vi "dosimat876_deliver.vi"(4 "error in":errorcluster, 6 "Volume":dbl format="%_4f", 7 "Dosimat Port In":refnum<visa-resource-name>="COM1") -> (0 "error out":errorcluster, 1 "Coerced?":bool, 2 "OutVolume":dbl, 3 "Dosimat Port Out":refnum<visa-resource-name>="COM1")   [LabVIEW 2010]
panel:
  # "Volume coerced!\nThe 876 will only accept volumes between 0.05 and 5.00 ml in increments of 0.05 ml. The volume has been changed to meet these requirements."
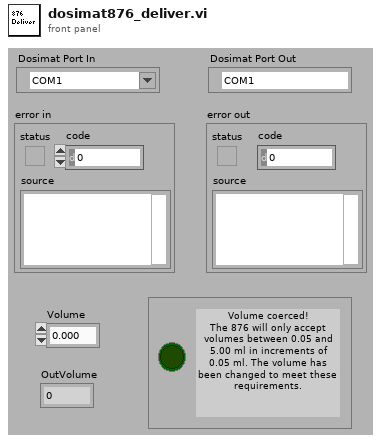
[diagram p1: front panel]
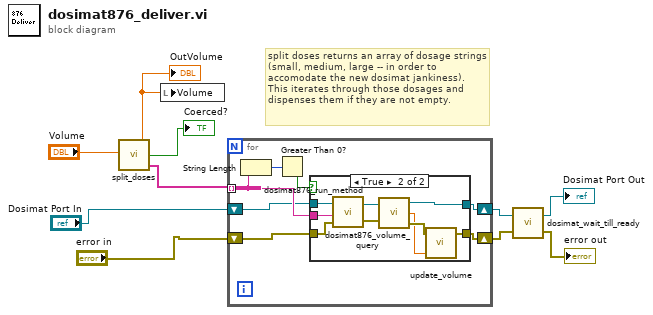
[diagram p0: block diagram]
diagram:
  # "split doses returns an array of dosage strings (small, medium, large -- in order to accomodate the new dosimat jankiness). This iterates through those dosages and dispenses them if they are not empty."
  n1 = call "split_doses.vi"("Volume"="Volume") -> ("Doses"=w7:string[], "Coerced?"=→"Coerced?":bool, "OutVolume"=w9:dbl)
  "OutVolume" <- w9
  n2 = local write "Volume"(w9) -> ()
  n3 = for {
    tunnel: w7 -> [w15] mode=indexing
    shift-right: [w12] -> w3
    shift-left: "Dosimat Port In" -> [w14]
    shift-right: [w11] -> w4
    shift-left: "error in" -> [w13]
    n4 = String Length(string=w15) -> (length=w17:i32)
    n5 = Greater Than 0?(x=w17) -> (x > 0?=w16:bool)
    n6 = case shown="True" w16 {
      tunnel: w15 -> [_ w27]
      tunnel: w14 -> [w19 w26]
      tunnel: [w19 w22] -> w12
      tunnel: [w18 w21] -> w11
      tunnel: w13 -> [w18 w25]
      frame False {
      }
      frame True {
        n7 = call "dosimat876_run_method.vi"("error in"=w25, "Method"=w27, "Dosimat Port In"=w26) -> ("error out"=w23:errorcluster, "Dosimat Port Out"=w24:refnum<visa-resource-name>)
        n8 = call "dosimat876_volume_query.vi"("error in"=w23, "Dosimat Port In"=w24) -> ("error out"=w21:errorcluster, "Volume"=w20:dbl, "Dosimat Port Out"=w22:refnum<visa-resource-name>)
        n9 = call "update_volume.vi"("Volume In"=w20) -> ()  [unwired: 1 in, 1 out]
      }
    }
  }
  n10 = call "dosimat_wait_till_ready.vi"("error in"=w4, "Dosimat Port In"=w3) -> ("error out"=→"error out":errorcluster, "Dosimat Port Out"=→"Dosimat Port Out":refnum<visa-resource-name>)
